vi "ZeroGyro.vi"(8 "error in":errorcluster) -> (0 "error out":errorcluster)   [LabVIEW 2016]
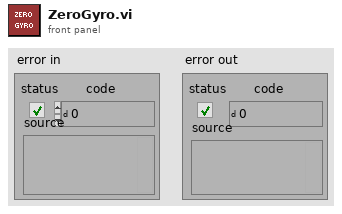
[diagram p1: front panel]
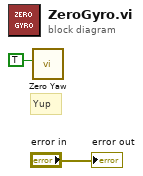
[diagram p0: block diagram]
diagram:
  # "Yup"
  n1 = call <vilib>:"Zero Yaw.vi"("Zero"=TRUE) -> ()  [unwired: 11 in]
  "error out" <- "error in"
